vi "Find Builds.vi"(10 "Project Path":path) -> (2 "Builds":T1[](array[typedef]) {"Last Update" format="%<%Y-%m-%d %H:%M:%S>T"})   [LabVIEW 2020, in "PicoG-Processor.lvlib" / "WebProjectWatcher.lvclass"]
uses:
  WebProjectWatcher.lvclass
  Web Build.ctl
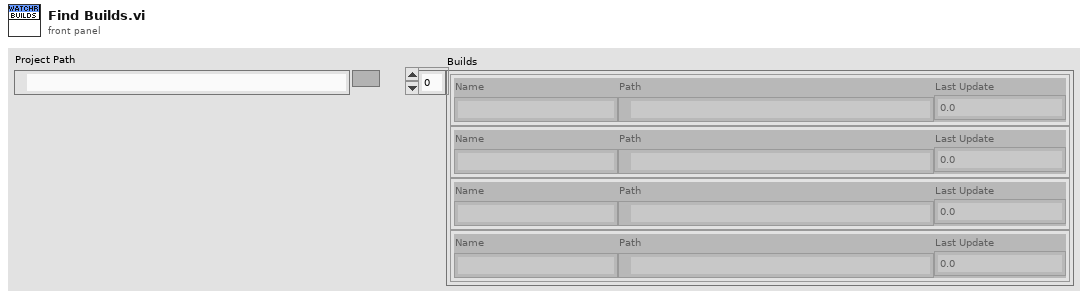
[diagram p1: front panel]
types:
  T1 = typedef "PicoG-Processor.lvlib/WebProjectWatcher.lvclass/Web Build.ctl" = cluster{"Name":string, "Path":path, "Last Update":dbl}
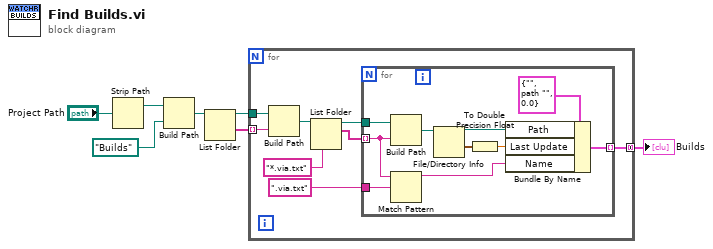
[diagram p0: block diagram]
diagram:
  n1 = Strip Path(path="Project Path") -> (stripped path=w6:path)  [unwired: 1 out]
  n2 = Build Path(base path=w6, name or relative path=path "Builds") -> (appended path=w4:path)
  n3 = List Folder(path=w4) -> (path out=w2:path, folder names=w3:string[])  [unwired: 3 in, 2 out]
  n4 = for {
    tunnel: w3 -> [w14] mode=indexing
    tunnel: w2 -> [w15]
    tunnel: [w8] -> w1 mode=concatenating
    n5 = Build Path(base path=w15, name or relative path=w14) -> (appended path=w13:path)
    n6 = List Folder(path=w13, pattern="*.via.txt") -> (path out=w11:path, filenames=w10:string[])  [unwired: 2 in, 2 out]
    n7 = for {
      tunnel: w11 -> [w25]
      tunnel: w10 -> [w24] mode=indexing
      tunnel: ".via.txt" ("pattern") -> [w23]
      tunnel: [w16] -> w8 mode=indexing
      n8 = Build Path(base path=w25, name or relative path=w24) -> (appended path=w22:path)
      n9 = Match Pattern(string=w24, regular expression=w23) -> (before substring=w19:string)  [unwired: 1 in, 3 out]
      n10 = File/Directory Info(path=w22) -> (path out=w17:path, last mod=w21:timestamp)  [unwired: 1 in, 5 out]
      n11 = To Double Precision Float(number=w21) -> (double precision float=w18:dbl)
      n12 = Bundle By Name(cluster=T1 {"Name"="", "Path"=path "", "Last Update"=0.0} ("Web Build"), "Path"=w17, "Last Update"=w18, "Name"=w19) -> (w16:T1)
    }
  }
  "Builds" <- w1
